vi "exercise3.vi"() -> ()   [LabVIEW 2025]
panel:
  in  "Numeric 3":dbl
  in  "Numeric 2":dbl
  in  "Numeric 1":dbl
  out "Plus Grande":ext
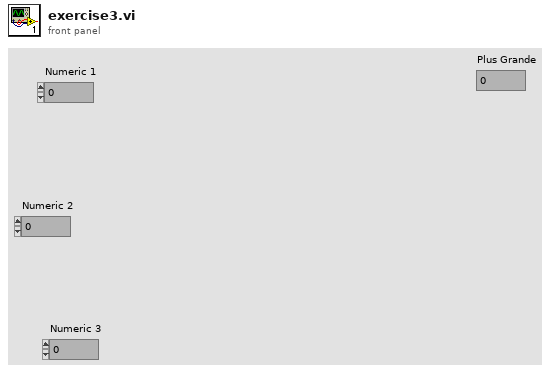
[diagram p1: front panel]
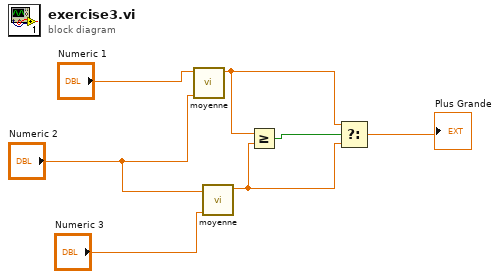
[diagram p0: block diagram]
diagram:
  n1 = call "moyenne.vi"("Y"="Numeric 2", "X"="Numeric 1") -> ("Moyenne"=w2:ext)  [unwired: 9 in]
  n2 = call "moyenne.vi"("Y"="Numeric 3", "X"="Numeric 2") -> ("Moyenne"=w1:ext)  [unwired: 9 in]
  n3 = Greater Or Equal?(x=w2, y=w1) -> (x >= y?=w3:bool)
  n4 = Select(t=w2, s=w3, f=w1) -> (s? t:f=→"Plus Grande":ext)
